vi "Get JSON Data.vi"(6 "Force Hide":bool, 7 "Evaluate Pane Move":bool, 8 "error in (no error)":errorcluster, 9 "Force Get All Data":bool, 10 "VI Reference":refnum<vi>, 11 "String In":refnum<class "Cluster.lvclass">) -> (0 "error out":errorcluster, 2 "JSON string":string, 3 "String Out":refnum<class "Cluster.lvclass">)   [LabVIEW 2017, in "Front Panel Publisher.lvlib" / "Cluster.lvclass"]
uses:
  Cluster.lvclass
  Control_class/Control.lvclass
  Object_class/Object.lvclass
  Web Front Panel_class/Controls/Enum - Control Display Mode.ctl
  Web Front Panel_class/Web Front Panel.lvclass
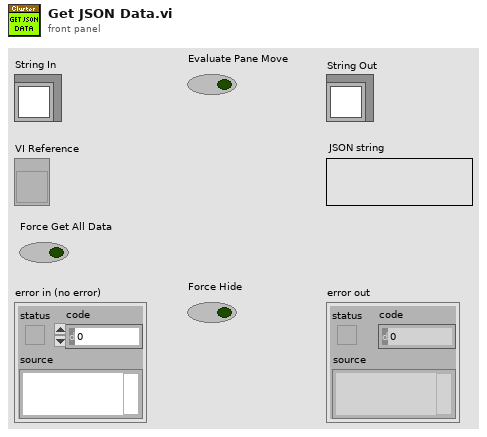
[diagram p1: front panel]
types:
  T1 = typedef "Front Panel Publisher.lvlib/Web Front Panel.lvclass/Enum - Control Display Mode.ctl" = enum16{"Value Only", "Value and Visibility", "Boolean Value Only", "Boolean Value and Visibility", "Control is Image", "Image and Visibility"}
  T2 = typedef "Front Panel Publisher.lvlib/Object.lvclass/Attributes.ctl" = cluster{"UID":i32, "Type":string, "Starting Location":T3, "Reference":refnum<vi>, "Cluster Component":bool, "Starting Rect Position":cluster{"Left":i16, "Top":i16}, "Owning Pane":refnum<vi>, "Master Total Rect Delta":T4}
  T3 = typedef "Front Panel Publisher.lvlib/Object.lvclass/Coordinates.ctl" = cluster{"Left":i32, "Top":i32, "Height":u32, "Width":u32}
  T4 = typedef "LVRectTypeDef.ctl" = cluster{"Left":i16, "Top":i16, "Right":i16, "Bottom":i16}
  T5 = typedef "Front Panel Publisher.lvlib/Control.lvclass/Attributes.ctl" = cluster{"Description":string, "Indicator":bool, "Default Value":variant, "Control Index":i32, "Label":refnum<class "Text.lvclass">, "Caption":refnum<class "Text.lvclass">, "Image b64":string, "No Control Index":bool, "Display Mode":T1}
  T6 = typedef "Front Panel Publisher.lvlib/Cluster.lvclass/Attributes.ctl" = cluster{"Cluster Decoration":refnum<class "Object.lvclass">, "Cluster Objects":refnum<class "Object.lvclass">[]}
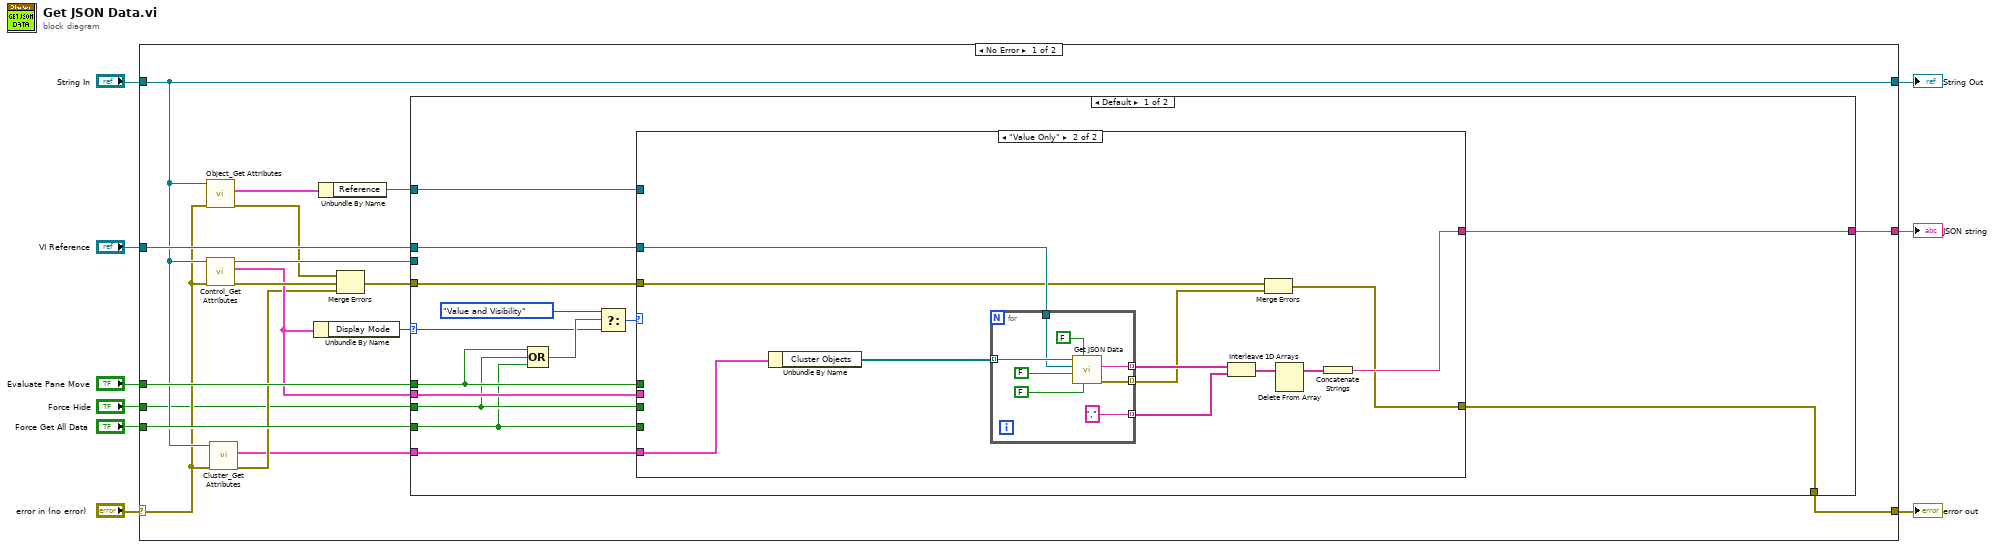
[diagram p0: block diagram]
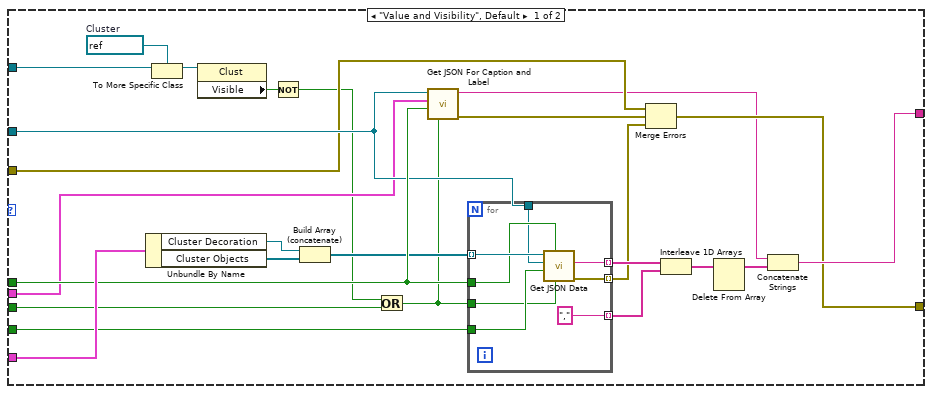
[diagram p2: hidden frame]
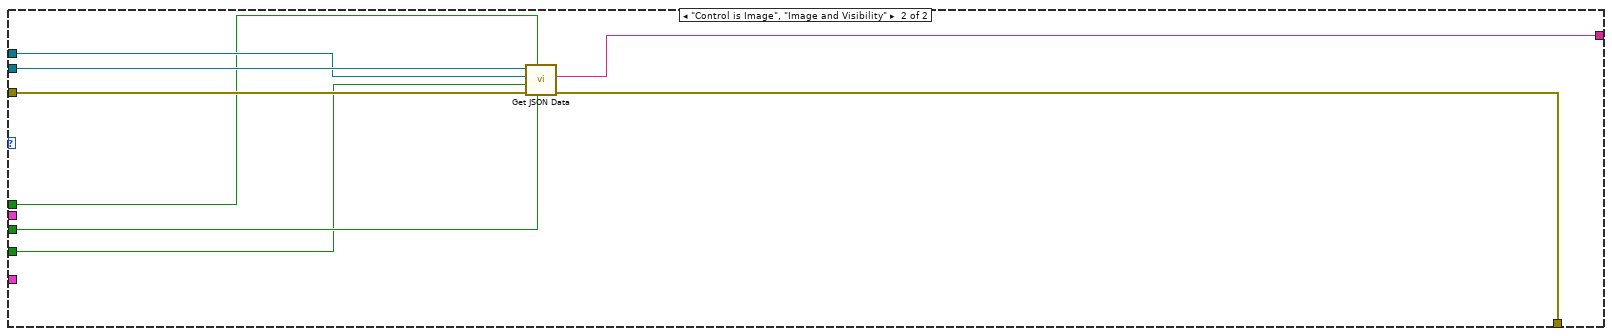
[diagram p3: hidden frame]
diagram:
  n1 = case shown="No Error" "error in (no error)" {
    selector: "error in (no error)" -> [w21 w103]
    tunnel: [w27 w103] -> w8
    tunnel: [w22 w102] -> w6
    tunnel: "String In" -> [w22 w102]
    tunnel: "VI Reference" -> [w26 _]
    tunnel: [w25 _] -> w4
    tunnel: "Force Get All Data" -> [w24 _]
    tunnel: "Evaluate Pane Move" -> [w23 _]
    tunnel: "Force Hide" -> [w10 _]
    frame No Error {
      n2 = call "Object_Get Attributes.vi"("error in (no error)"=w21, "Object In"=w22) -> ("error out"=w14:errorcluster, "Object Attributes"=w19:T2)  [unwired: 7 in, 1 out]
      n3 = call "Control_Get Attributes.vi"("error in (no error)"=w21, "Control In"=w22) -> ("error out"=w20:errorcluster, "Control Attributes"=w13:T5, "Control Out"=w17:refnum<class "Cluster.lvclass">)  [unwired: 7 in]
      n4 = call "Cluster_Get Attributes.vi"("error in (no error)"=w21, "Cluster In"=w22) -> ("error out"=w12:errorcluster, "Cluster Attributes"=w11:T6)  [unwired: 7 in, 1 out]
      n5 = Unbundle By Name(w13) -> ("Display Mode"=w18:T1)
      n6 = Unbundle By Name(w19) -> ("Reference"=w16:refnum<vi>)
      n7 = Merge Errors(w14, w20, w12) -> (w15:errorcluster)
      n8 = case shown="Default" w18 {
        selector: w18 -> [w32 _]
        tunnel: w15 -> [w37 w99]
        tunnel: [w36 w98] -> w27
        tunnel: w26 -> [w40 w100]
        tunnel: [w39 w97] -> w25
        tunnel: w17 -> [_ w101]
        tunnel: w16 -> [w38 _]
        tunnel: w13 -> [w35 _]
        tunnel: w24 -> [w28 w94]
        tunnel: w23 -> [w31 w96]
        tunnel: w11 -> [w41 _]
        tunnel: w10 -> [w29 w95]
        frame Default {
          n9 = Compound Arithmetic op=OR(w31, w29, w28) -> (w33:bool)
          n10 = Select(t=Enum_-_Control_Display_Mode."Value and Visibility", s=w33, f=w32) -> (s? t:f=w30:T1)
          n11 = case shown="\"Value Only\"" w30 {
            tunnel: w41 -> [w66 w85]
            tunnel: w31 -> [w65 _]
            tunnel: w40 -> [w64 w84]
            tunnel: w28 -> [w63 _]
            tunnel: [w62 w83] -> w39
            tunnel: w38 -> [w61 _]
            tunnel: w37 -> [w60 w82]
            tunnel: [w59 w81] -> w36
            tunnel: w35 -> [w58 _]
            tunnel: w29 -> [w57 _]
            frame "Value and Visibility", Default {
              w47 = refnum<vi> refnum  # Cluster
              n12 = Unbundle By Name(w66) -> ("Cluster Decoration"=w56:refnum<class "Object.lvclass">, "Cluster Objects"=w55:refnum<class "Object.lvclass">[])
              n13 = To More Specific Class(target class=w47, reference=w61) -> (specific class reference=w48:refnum<vi>)  [unwired: 1 in, 1 out]
              n14 = property class="Clust"(reference=w48) -> ("Visible"=w46:bool)  [unwired: 1 in, 2 out]
              n15 = Not(x=w46) -> (.not. x?=w45:bool)
              n16 = Build Array (concatenate)(w56, w55) -> (w54:refnum<class "Object.lvclass">[])
              n17 = Or(x=w45, y=w57) -> (x .or. y?=w44:bool)
              n18 = call "Get JSON For Caption and Label.vi"("Force Hide"=w44, "Evaluate Pane Move"=w65, "Data"=w58, "VI in"=w64) -> ("error out"=w42:errorcluster, "JSON"=w49:string)  [unwired: 6 in]
              n19 = for {
                tunnel: w54 -> [w74] mode=indexing
                tunnel: w65 -> [w73]
                tunnel: w64 -> [w72]
                tunnel: w63 -> [w71]
                tunnel: [w70] -> w53 mode=indexing
                tunnel: [","] -> w52 mode=indexing
                tunnel: w44 -> [w68]
                tunnel: [w67] -> w43 mode=indexing
                n20 = call-dynamic "Get JSON Data.vi"("Force Hide"=w68, "Evaluate Pane Move"=w73, "Force Get All Data"=w71, "VI Reference"=w72, "Object In"=w74) -> ("error out"=w67:errorcluster, "JSON string"=w70:string)  [unwired: 4 in, 1 out]
              }
              n21 = Merge Errors(w60, w42, w43) -> (w59:errorcluster)
              n22 = Interleave 1D Arrays(w53, w52) -> (w50:string[])
              n23 = Delete From Array(array=w50) -> (array with subset deleted=w51:string[])  [unwired: 2 in, 1 out]
              n24 = Concatenate Strings(w49, w51) -> (w62:string)
            }
            frame "Value Only" {
              n25 = Unbundle By Name(w85) -> ("Cluster Objects"=w75:refnum<class "Object.lvclass">[])
              n26 = for {
                tunnel: w75 -> [w93] mode=indexing
                tunnel: w84 -> [w92]
                tunnel: [w91] -> w80 mode=indexing
                tunnel: [","] -> w79 mode=indexing
                tunnel: [w89] -> w76 mode=indexing
                n27 = call-dynamic "Get JSON Data.vi"("Force Hide"=FALSE, "Evaluate Pane Move"=FALSE, "Force Get All Data"=FALSE, "VI Reference"=w92, "Object In"=w93) -> ("error out"=w89:errorcluster, "JSON string"=w91:string)  [unwired: 4 in, 1 out]
              }
              n28 = Interleave 1D Arrays(w80, w79) -> (w77:string[])
              n29 = Merge Errors(w82, w76) -> (w81:errorcluster)
              n30 = Delete From Array(array=w77) -> (array with subset deleted=w78:string[])  [unwired: 2 in, 1 out]
              n31 = Concatenate Strings(w78) -> (w83:string)
            }
          }
        }
        frame "Control is Image", "Image and Visibility" {
          n32 = call-parent "Get JSON Data.vi"("Force Hide"=w95, "Evaluate Pane Move"=w96, "error in (no error)"=w99, "Force Get All Data"=w94, "VI Reference"=w100, "Control In"=w101) -> ("error out"=w98:errorcluster, "JSON string"=w97:string)  [unwired: 3 in, 1 out]
        }
      }
    }
    frame Error {
    }
  }
  "error out" <- w8
  "String Out" <- w6
  "JSON string" <- w4
